vi "Plantita old.vi"() -> ()   [LabVIEW 2019]
uses:
  plantitaStates.ctl
  <vilib>/addons/control/pid/pid.llb/PID (DBL).vi
  <vilib>/addons/control/pid/NI_PID_pid.lvlib
panel:
  in  "Turbidity":bool
  in  "Sludge control":bool
  in  "Sludge valve [V]":dbl(slide)=1.5 scale=0.0..5.0
  in  "Coagulant  [V]":dbl(slide)=0.3 scale=0.0..5.0
  in  "Coagulant control":bool
  in  "Main valve [V]":dbl(slide)=2.5 scale=0.0..5.0
  in  "Flow control":bool
  out "Main valve":dbl(graph)
  in  "Shut Down":bool
  out "22 [NTU]":dbl
  out "Save File Path 2":path=path "C:/1.tdms"
  out "Settled [NTU]":dbl
  out "23 [NTU]":dbl
  out "21 [NTU]":dbl
  in  "Ripen time [s]":dbl=600.0
  in  "Backwash time [s]":dbl=600.0
  out "Last backwash":timestamp
  in  "Filtered quality target [NTU]":dbl=0.3
  out "Coagulant [mg Al/L]":dbl(graph)
  in  "Coagulant PID gains":T1={"proportional gain (Kc)"=-0.1, "integral time (Ti, min)"=33.0, "derivative time (Td, min)"=6.5} {"derivative time (Td, min)" format="%.3f"; "integral time (Ti, min)" format="%.3f"; "proportional gain (Kc)" format="%.3f"}
  out "Turbidities":dbl[][](graph)
  in  "Backwash control":bool
  out "UV 254":dbl[][](graph)
  in  "Sludge flow [L/min]":dbl=0.84
  in  "Sludge PID gains":T1={"proportional gain (Kc)"=0.07, "integral time (Ti, min)"=1.0, "derivative time (Td, min)"=0.01} {"derivative time (Td, min)" format="%.3f"; "integral time (Ti, min)" format="%.3f"; "proportional gain (Kc)" format="%.3f"}
  in  "Main PID gains":T1={"proportional gain (Kc)"=0.05, "integral time (Ti, min)"=1.0, "derivative time (Td, min)"=0.01} {"derivative time (Td, min)" format="%.3f"; "integral time (Ti, min)" format="%.3f"; "proportional gain (Kc)" format="%.3f"}
  in  "Main flow [L/min]":dbl=30.0
  out "Filter head loss":dbl
  out "Water flow value":dbl
  out "Sludge flow value":dbl
  in  "Settled quality target [NTU]":dbl=0.3
  in  "backwash [ON/OFF]":bool
  out "Sludge valve":dbl(graph)
  out "Sludge flow meter":dbl[][](graph)
  out "Filter head loss":dbl[][](graph)
  out "Main flow meter":dbl[][](graph)
  out "error out":errorcluster
  in  "Input: Seconds per data point (sec)":dbl=1.0
  in  "Start Experiment":bool
  in  "Exit":bool
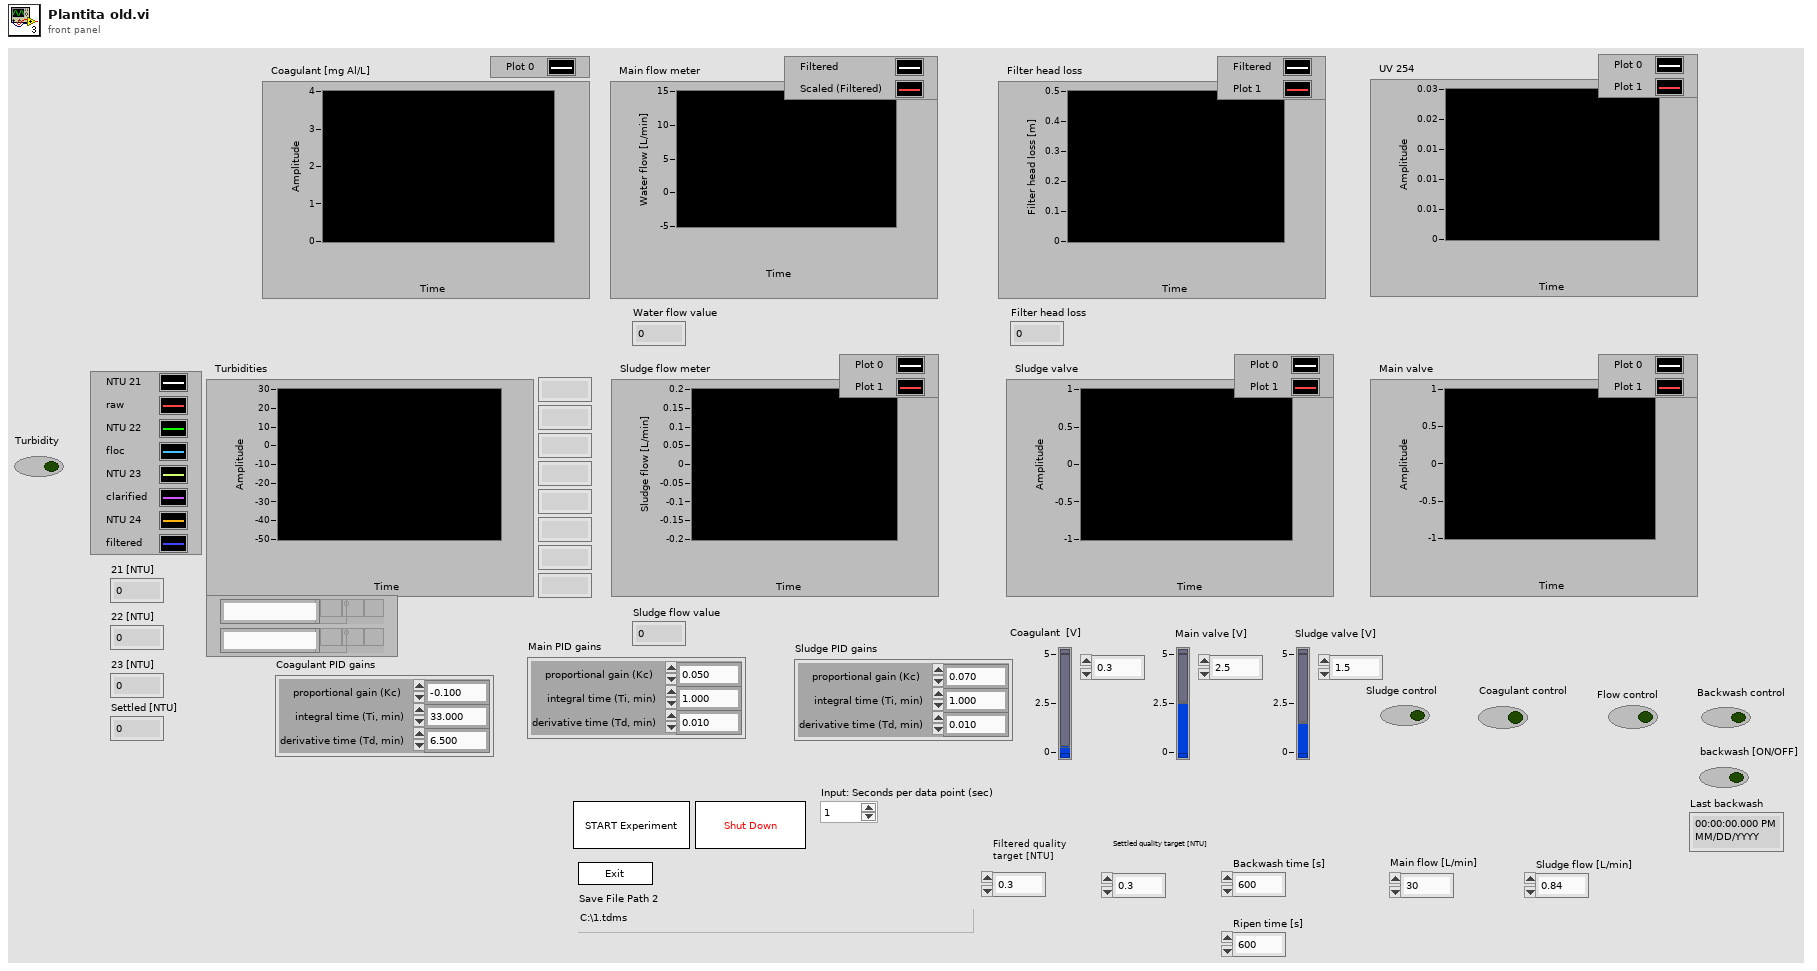
[diagram p1: front panel]
types:
  T1 = cluster{"proportional gain (Kc)":dbl, "integral time (Ti, min)":dbl, "derivative time (Td, min)":dbl}
  T2 = cluster{"Boolean <Replace Me>":bool, "String <Replace Me>":string, "Numeric <Replace Me>":dbl}
  T3 = typedef "plantitaStates.ctl" = enum16{"Initialize", "Wait for Event", "Experiment", "Exit"}
  T4 = enum16{"open", "open or create", "create or replace", "create", "open (read-only)"}
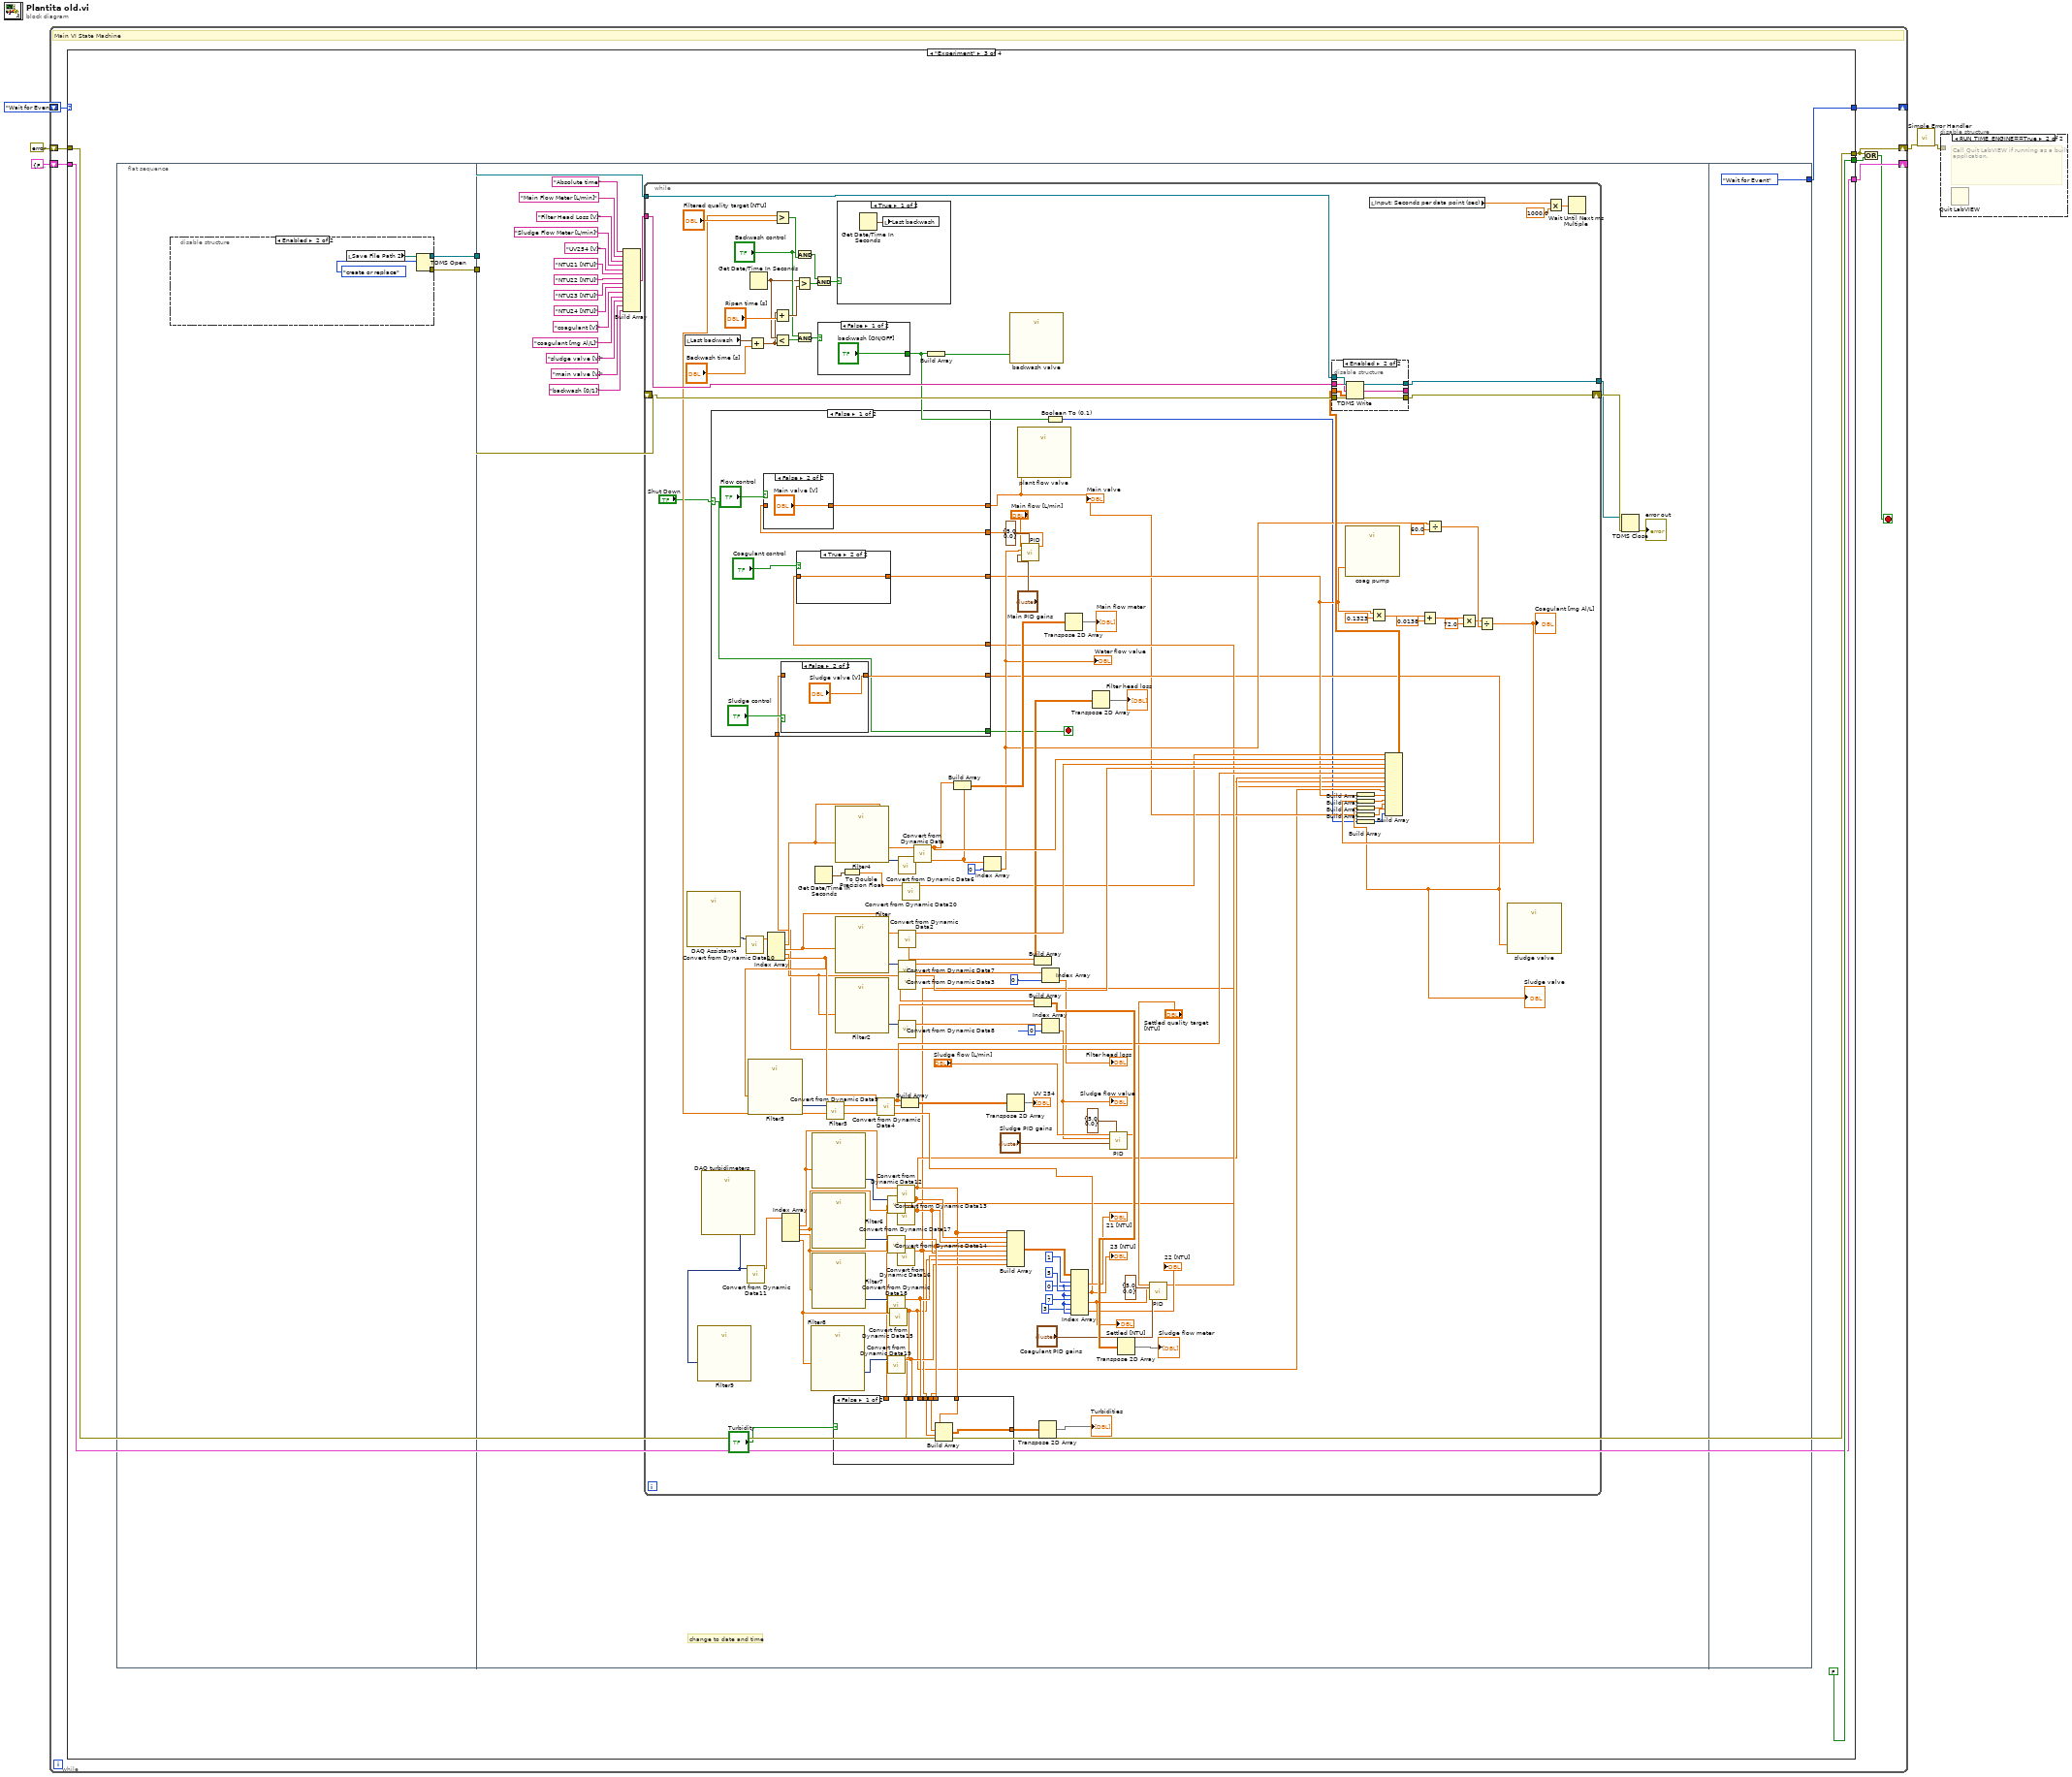
[diagram p0: block diagram]
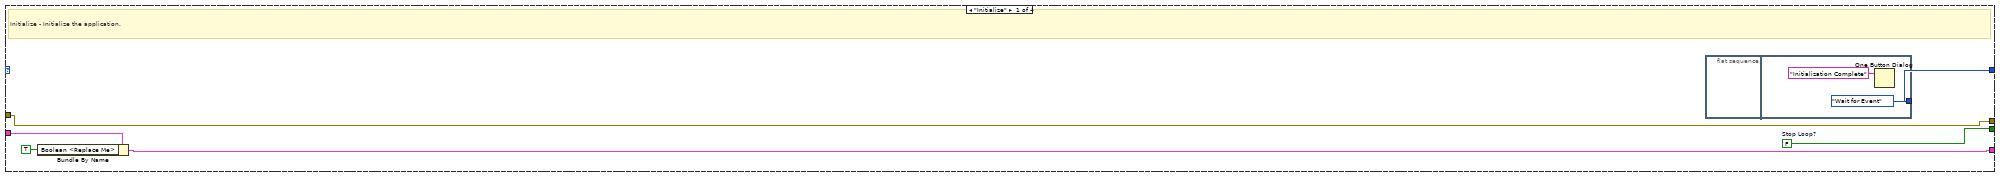
[diagram p3: hidden frame]
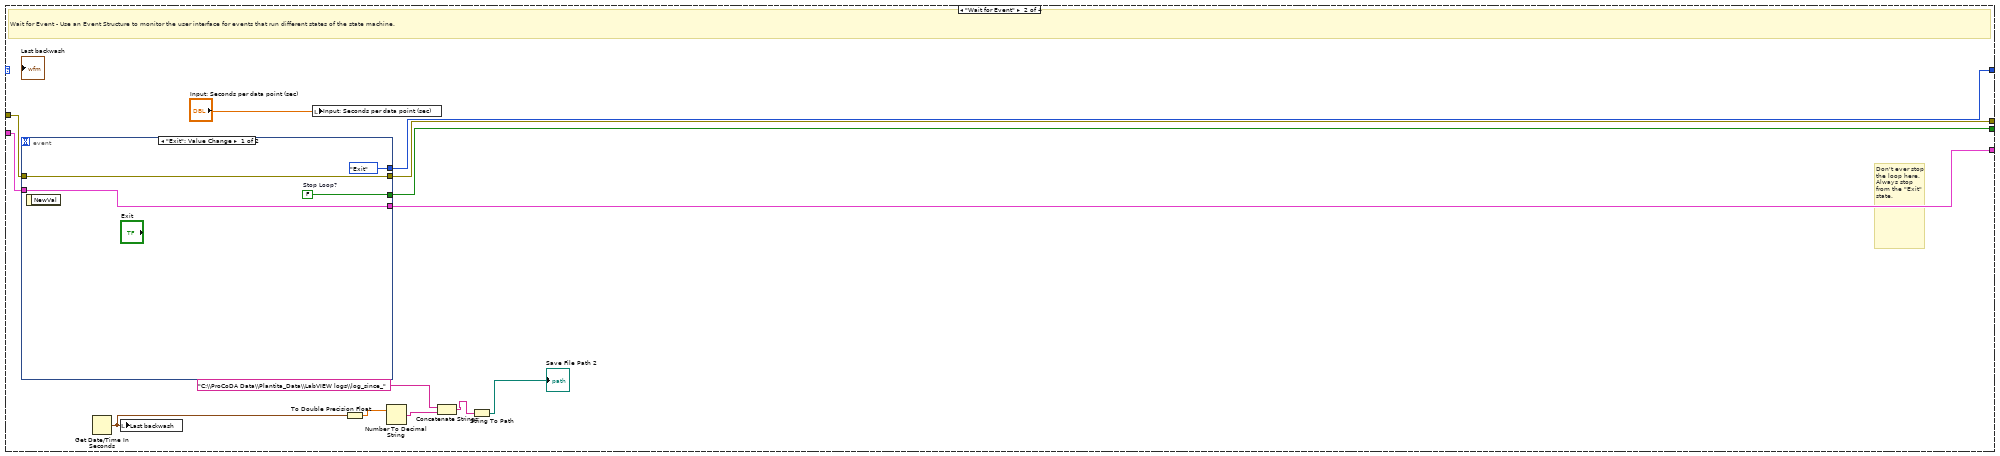
[diagram p4: hidden frame]
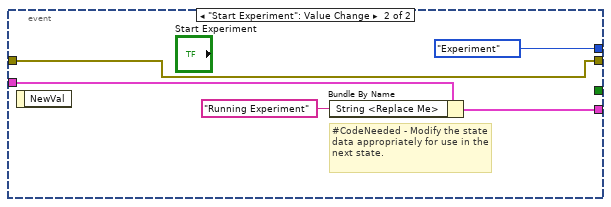
[diagram p5: hidden frame]
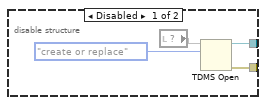
[diagram p6: hidden frame]
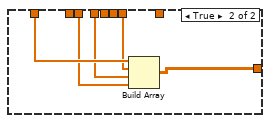
[diagram p7: hidden frame]
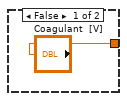
[diagram p9: hidden frame]
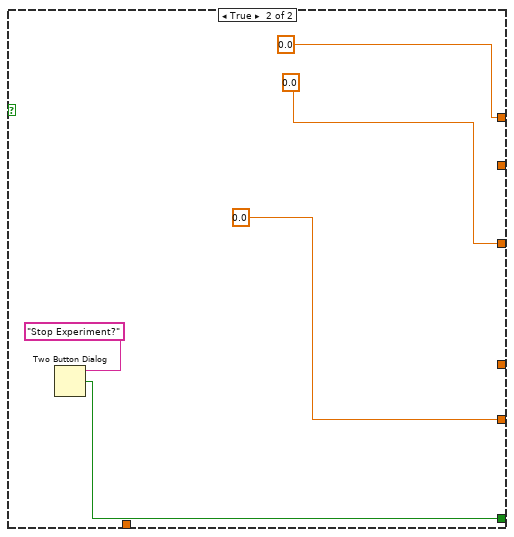
[diagram p11: hidden frame]
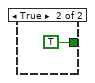
[diagram p12: hidden frame]
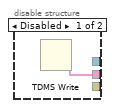
[diagram p14: hidden frame]
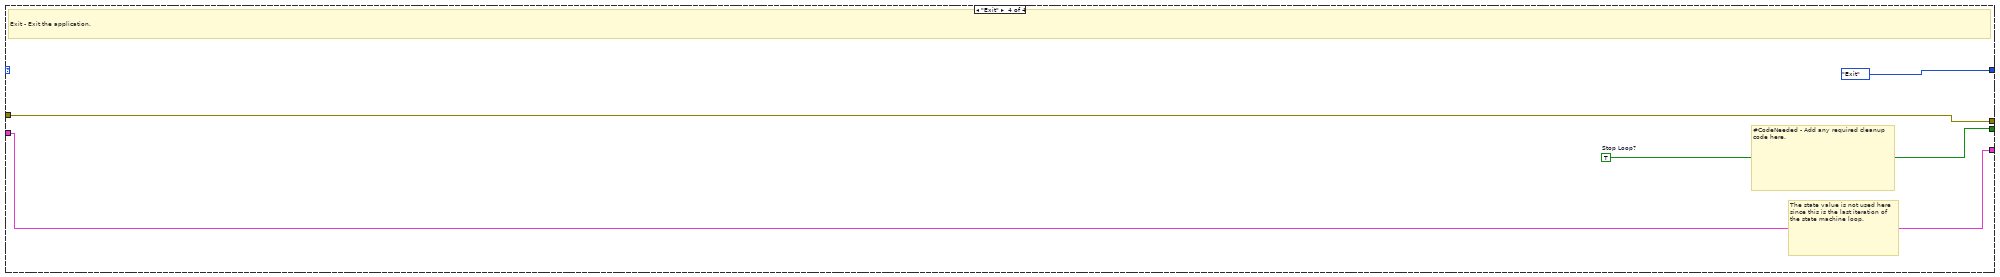
[diagram p15: hidden frame]
diagram:
  n1 = while {
    shift-right: [w12] -> _
    shift-left: plantitaStates."Wait for Event" ("Initial State") -> [w13]
    shift-right: [w10] -> _
    shift-left: T2 {"Boolean <Replace Me>"=FALSE, "String <Replace Me>"="", "Numeric <Replace Me>"=0.0} -> [w11]
    shift-right: [w6] -> w3
    shift-left: errorcluster {"status"=FALSE, "code"=0, "source"=""} ("error constant") -> [w9]
    stop <- w7 stop-if-true
    # "Main VI State Machine"
    n2 = case shown="\"Experiment\"" w13 {
      tunnel: [w14 w34 w46 plantitaStates."Exit" ("(Value Not Used)")] -> w12
      tunnel: [w19 w29 FALSE ("Stop Loop?") w252] -> w8
      tunnel: w11 -> [w18 w33 w48 w253]
      tunnel: [w17 w32 w48 w253] -> w10
      tunnel: w9 -> [w15 w31 w47 w251]
      tunnel: [w15 w30 w47 w251] -> w6
      frame "Initialize" {
        w19 = FALSE  # Stop Loop?
        # "Initialize - Initialize the application."
        n3 = Bundle By Name(cluster=w18, "Boolean <Replace Me>"=TRUE ("Replace_Me_Boolean")) -> (w17:T2)
        n4 = flat-sequence {
          tunnel: [plantitaStates."Wait for Event" ("Next State")] -> w14
          frame #0 {
          }
          frame #1 {
            n5 = One Button Dialog(message="Initialization Complete") -> ()  [unwired: 1 in, 1 out]
          }
        }
      }
      frame "Wait for Event" {
        # "Don't ever stop the loop here. Always stop from the \"Exit\" state."
        # "Wait for Event - Use an Event Structure to monitor the user interface for events that run different states of the state machine."
        n6 = event shown="[0] \"Exit\": Value Change" {
          selector: _ -> [_ _]
          dyn-events: _ -> [_ _]
          timeout: _ -> [_ _]
          tunnel: [plantitaStates."Exit" ("Next State") plantitaStates."Experiment" ("Next State")] -> w34
          tunnel: w33 -> [w37 w42]
          tunnel: [w37 w41] -> w32
          tunnel: w31 -> [w36 w39]
          tunnel: [w36 w39] -> w30
          tunnel: [w35 _] -> w29
          event "Exit": Value Change {
            w35 = FALSE  # Stop Loop?
            n7 = event-data() -> ()  [unwired: 1 in, 1 out]
          }
          event "Start Experiment": Value Change {
            # "#CodeNeeded - Modify the state data appropriately for use in the next state."
            n8 = event-data() -> ()  [unwired: 1 in, 1 out]
            n9 = Bundle By Name(cluster=w42, "String <Replace Me>"="Running Experiment" ("Running User State 1")) -> (w41:T2)
          }
        }
        n10 = Get Date/Time In Seconds() -> (seconds since 1Jan1904=w27:timestamp)
        n11 = local write "Last backwash"(w27) -> ()
        n12 = local write "Input: Seconds per data point (sec)"("Input: Seconds per data point (sec)") -> ()
        n13 = To Double Precision Float(number=w27) -> (double precision float=w25:dbl)
        n14 = Number To Decimal String(number=w25) -> (decimal integer string=w24:string)  [unwired: 1 in]
        n15 = Concatenate Strings("C:\\ProCoDA Data\\Plantita_Data\\LabVIEW logs\\log_since_", w24) -> (w23:string)
        n16 = String To Path(string=w23) -> (path=→"Save File Path 2":path)
      }
      frame "Experiment" {
        n17 = flat-sequence {
          tunnel: [w51] -> w45
          tunnel: [w50] -> w44
          tunnel: w45 -> [w77]
          tunnel: w44 -> [w79]
          tunnel: [plantitaStates."Wait for Event" ("Next State")] -> w46
          frame #0 {
            n18 = disable-structure shown="Enabled" {
              disable-tunnel: [w55 w57] -> w51
              disable-tunnel: [w54 w56] -> w50
              frame Disabled {
                n19 = local read item#-1() -> (w53)
                n20 = TDMS Open(10:T4."create or replace" ("operation (0:open)"), 11:w53) -> (0:w54:errorcluster, 3:w55:refnum<k34>)  [unwired: 5 in]
              }
              frame Enabled {
                n21 = local read "Save File Path 2"() -> (w59:path)
                n22 = TDMS Open(10:T4."create or replace" ("operation (0:open)"), 11:w59) -> (0:w56:errorcluster, 3:w57:refnum<k34>)  [unwired: 5 in]
              }
            }
          }
          frame #1 {
            # "change to date and time"
            n23 = Build Array("Absolute time", "Main Flow Meter [L/min]", "Filter Head Loss [V]", "Sludge Flow Meter [L/min]", "UV254 [V]" ("element"), "NTU21 [NTU]", "NTU22 [NTU]", "NTU23 [NTU]", "NTU24 [NTU]" ("element"), "coagulant [V]" ("element"), "coagulant [mg Al/L]" ("element"), "sludge valve [V]" ("element"), "main valve [V]" ("element"), "backwash [0/1]" ("element")) -> (w78:string[])
            n24 = while {
              shift-right: [w196] -> w75
              shift-left: w79 -> [w199]
              tunnel: w78 -> [w197]
              tunnel: w77 -> [w198]
              tunnel: [w195] -> w74
              stop <- w93 stop-if-true
              w103 = 0 ("disabled index (col)")
              n25 = local read "Last backwash"() -> (w132:timestamp)
              n26 = call "DAQ Assistant4"() -> ("data"=w168:dynamicdata)  [unwired: 17 in, 2 out]
              n27 = call "DAQ turbidimeters"() -> ("data"=w80:dynamicdata)  [unwired: 17 in, 2 out]
              n28 = call "Filter9"("Signal"=w80) -> ()  [unwired: 9 in, 2 out]
              n29 = call "Convert from Dynamic Data10"("Dynamic Data Type"=w168) -> ("Array"=w169:dbl[])  [unwired: 3 in]
              n30 = call "Convert from Dynamic Data11"("Dynamic Data Type"=w80) -> ("Array"=w159:dbl[])  [unwired: 3 in]
              n31 = Add(x=w132, y="Backwash time [s]") -> (x+y=w122:timestamp)
              n32 = Get Date/Time In Seconds() -> (seconds since 1Jan1904=w123:timestamp)
              n33 = Index Array(array=w169) -> (element #1=w167:dbl, element #2=w162:dbl, element #3=w166:dbl, element #4=w170:dbl)  [unwired: 4 in]
              n34 = call "Filter3"("Signal"=w170) -> ("Filtered Signal"=w184:dynamicdata)  [unwired: 9 in, 1 out]
              n35 = Add(x=w122, y="Ripen time [s]") -> (x+y=w130:timestamp)
              n36 = Less?(x=w123, y=w122) -> (x < y?=w124:bool)
              n37 = Index Array(array=w159) -> (element #1=w158:dbl, element #2=w154:dbl, element #3=w152:dbl, element #4=w147:dbl)  [unwired: 4 in]
              n38 = Greater?(x=w123, y=w130) -> (0:w128:bool)
              n39 = And(x="Backwash control", y=w124) -> (x .and. y?=w121:bool)
              n40 = call "Filter8"("Signal"=w147) -> ("Filtered Signal"=w148:dynamicdata)  [unwired: 9 in, 1 out]
              n41 = call "Filter5"("Signal"=w158) -> ("Filtered Signal"=w157:dynamicdata)  [unwired: 9 in, 1 out]
              n42 = call "Filter6"("Signal"=w154) -> ("Filtered Signal"=w153:dynamicdata)  [unwired: 9 in, 1 out]
              n43 = call "Filter7"("Signal"=w152) -> ("Filtered Signal"=w149:dynamicdata)  [unwired: 9 in, 1 out]
              n44 = Get Date/Time In Seconds() -> (seconds since 1Jan1904=w151:timestamp)
              n45 = case shown="False" w121 {
                tunnel: ["backwash [ON/OFF]" TRUE ("backwash [ON/OFF]")] -> w111
                frame False {
                }
                frame True {
                }
              }
              n46 = call "Convert from Dynamic Data9"("Dynamic Data Type"=w184) -> ("Array"=w179:dbl[])  [unwired: 3 in]
              n47 = call "Filter4"("Signal"=w167) -> ("Filtered Signal"=w193:dynamicdata)  [unwired: 9 in, 1 out]
              n48 = call "Filter"("Signal"=w162) -> ("Filtered Signal"=w188:dynamicdata)  [unwired: 9 in, 1 out]
              n49 = call "Filter2"("Signal"=w166) -> ("Filtered Signal"=w185:dynamicdata)  [unwired: 9 in, 1 out]
              n50 = To Double Precision Float(number=w151) -> (double precision float=w150:dbl)
              n51 = call "Convert from Dynamic Data4"("Dynamic Data Type"=w170) -> ("Array"=w180:dbl[])  [unwired: 3 in]
              n52 = call "Convert from Dynamic Data13"("Dynamic Data Type"=w157) -> ("Array"=w91:dbl[])  [unwired: 3 in]
              n53 = call "Convert from Dynamic Data14"("Dynamic Data Type"=w153) -> ("Array"=w90:dbl[])  [unwired: 3 in]
              n54 = call "Convert from Dynamic Data18"("Dynamic Data Type"=w149) -> ("Array"=w89:dbl[])  [unwired: 3 in]
              n55 = call "Convert from Dynamic Data19"("Dynamic Data Type"=w148) -> ("Array"=w88:dbl[])  [unwired: 3 in]
              n56 = call "Convert from Dynamic Data15"("Dynamic Data Type"=w147) -> ("Array"=w84:dbl[])  [unwired: 3 in]
              n57 = call "Convert from Dynamic Data12"("Dynamic Data Type"=w158) -> ("Array"=w87:dbl[])  [unwired: 3 in]
              n58 = call "Convert from Dynamic Data17"("Dynamic Data Type"=w154) -> ("Array"=w86:dbl[])  [unwired: 3 in]
              n59 = call "Convert from Dynamic Data16"("Dynamic Data Type"=w152) -> ("Array"=w85:dbl[])  [unwired: 3 in]
              n60 = case shown="False" "Turbidity" {
                tunnel: [w207 w212] -> w92
                tunnel: w91 -> [_ w211]
                tunnel: w90 -> [_ w210]
                tunnel: w89 -> [_ w209]
                tunnel: w88 -> [_ w208]
                tunnel: w87 -> [w206 _]
                tunnel: w86 -> [w205 _]
                tunnel: w85 -> [w204 _]
                tunnel: w84 -> [w203 _]
                frame False {
                  n61 = Build Array "Build Array"(w206, w205, w204, w203) -> (w207:dbl[][])
                }
                frame True {
                  n62 = Build Array "Build Array"(w211, w210, w209, w208) -> (w212:dbl[][])
                }
              }
              n63 = call "Convert from Dynamic Data6"("Dynamic Data Type"=w193) -> ("Array"=w177:dbl[])  [unwired: 3 in]
              n64 = call "Convert from Dynamic Data7"("Dynamic Data Type"=w188) -> ("Array"=w172:dbl[])  [unwired: 3 in]
              n65 = call "Convert from Dynamic Data8"("Dynamic Data Type"=w185) -> ("Array"=w171:dbl[])  [unwired: 3 in]
              n66 = call "Convert from Dynamic Data2"("Dynamic Data Type"=w162) -> ("Array"=w189:dbl[])  [unwired: 3 in]
              n67 = call "Convert from Dynamic Data3"("Dynamic Data Type"=w166) -> ("Array"=w183:dbl[])  [unwired: 3 in]
              n68 = Build Array(w180, w179) -> (w178:dbl[][])
              n69 = call "Convert from Dynamic Data20"("Dynamic Data Type"=w150) -> ("Array"=w109:dbl[])  [unwired: 3 in]
              n70 = call "Convert from Dynamic Data"("Dynamic Data Type"=w167) -> ("Array"=w190:dbl[])  [unwired: 3 in]
              n71 = Build Array(w111) -> (w112:bool[])
              n72 = Build Array(w190, w177) -> (w191:dbl[][])
              n73 = Index Array(array=w177, index=0) -> (element=w139:dbl)
              "Water flow value" <- w139
              n74 = Transpose 2D Array(2D array=w178) -> (transposed array=→"UV 254":dbl[][])
              n75 = Build Array "Build Array"(w87, w91, w86, w90, w85, w89, w84, w88) -> (w120:dbl[][])
              n76 = call "backwash valve"("data"=w112) -> ()  [unwired: 17 in, 2 out]
              n77 = call-poly <vilib>:"PID.vi"("output range"=cluster{"output high":dbl, "output low":dbl} {"output high"=5.0, "output low"=0.0}, "PID gains"="Main PID gains", "process variable"=w139, "setpoint"="Main flow [L/min]") -> ("output"=w99:dbl)  [unwired: 6 in, 1 out]
              n78 = Build Array(w189, w172) -> (w186:dbl[][])
              n79 = Build Array(w183, w171) -> (w182:dbl[][])
              n80 = Transpose 2D Array(2D array=w92) -> (transposed array=→"Turbidities":dbl[][])
              n81 = Index Array(array=w172, index=0) -> (element=→"Filter head loss":dbl)
              n82 = Index Array(array=w171, index=0) -> (element=w156:dbl)
              "Sludge flow value" <- w156
              n83 = Boolean To (0,1)(Boolean=w111) -> (0, 1=w81:i16)
              n84 = Transpose 2D Array(2D array=w191) -> (transposed array=→"Main flow meter":dbl[][])
              n85 = Index Array(array=w120, index (row) #1=1 ("index (row)"), index (col) #1=w103, index (row) #2=5 ("disabled index (row)"), index (col) #2=w103, index (row) #3=7 ("disabled index (row)"), index (col) #3=w103, index (row) #4=3 ("disabled index (row)"), index (col) #4=w103) -> (element #1=→"21 [NTU]":dbl, element #2=w113:dbl, element #3=w115:dbl, element #4=→"22 [NTU]":dbl)
              "23 [NTU]" <- w113
              "Settled [NTU]" <- w115
              n86 = Greater?(x=w113, y="Filtered quality target [NTU]") -> (0:w134:bool)
              n87 = And(x="Backwash control", y=w134) -> (x .and. y?=w126:bool)
              n88 = And(x=w126, y=w128) -> (x .and. y?=w127:bool)
              n89 = case shown="True" w127 {
                frame True {
                  n90 = Get Date/Time In Seconds() -> (seconds since 1Jan1904=w236:timestamp)
                  n91 = local write "Last backwash"(w236) -> ()
                }
                frame False {
                }
              }
              n92 = Transpose 2D Array(2D array=w186) -> (transposed array=→"Filter head loss":dbl[][])
              n93 = call-poly <vilib>:"PID.vi"("output range"=cluster{"output high":dbl, "output low":dbl} {"output high"=5.0, "output low"=0.0}, "PID gains"="Sludge PID gains", "process variable"=w156, "setpoint"="Sludge flow [L/min]") -> ("output"=w96:dbl)  [unwired: 6 in, 1 out]
              n94 = Transpose 2D Array(2D array=w182) -> (transposed array=→"Sludge flow meter":dbl[][])
              n95 = call-poly <vilib>:"PID.vi"("output range"=cluster{"output high":dbl, "output low":dbl} {"output high"=5.0, "output low"=0.0}, "PID gains"="Coagulant PID gains", "process variable"=w115, "setpoint"="Settled quality target [NTU]") -> ("output"=w97:dbl)  [unwired: 6 in, 1 out]
              n96 = case shown="False" "Shut Down" {
                selector: "Shut Down" -> [w213 _]
                tunnel: w99 -> [w221 _]
                tunnel: [w220 0.0 ("Main valve [V] 2")] -> w94
                tunnel: [w218 0.0 ("Main valve [V] 2")] -> w98
                tunnel: w97 -> [w217 _]
                tunnel: w96 -> [w215 _]
                tunnel: [w214 0.0 ("Main valve [V] 2")] -> w95
                tunnel: [w213 w229] -> w93
                frame False {
                  n97 = case shown="False" "Flow control" {
                    tunnel: [w227 "Main valve [V]"] -> w220
                    tunnel: w221 -> [w227 _]
                    frame True {
                    }
                    frame False {
                    }
                  }
                  n98 = case shown="False" "Sludge control" {
                    tunnel: [w223 "Sludge valve [V]"] -> w214
                    tunnel: w215 -> [w223 _]
                    frame True {
                    }
                    frame False {
                    }
                  }
                  n99 = case shown="True" "Coagulant control" {
                    tunnel: w217 -> [_ w226]
                    tunnel: ["Coagulant  [V]" w226] -> w218
                    frame False {
                    }
                    frame True {
                    }
                  }
                }
                frame True {
                  n100 = Two Button Dialog(message="Stop Experiment?") -> (T button?=w229:bool)  [unwired: 2 in]
                }
              }
              "Sludge valve" <- w95
              "Main valve" <- w94
              n101 = call "plant flow valve"("data"=w94) -> ()  [unwired: 17 in, 2 out]
              n102 = call "coag pump"("data"=w98) -> ()  [unwired: 17 in, 2 out]
              n103 = Build Array(w98) -> (w104:dbl[])
              n104 = Build Array(w95) -> (w106:dbl[])
              n105 = Build Array(w94) -> (w107:dbl[])
              n106 = Build Array(w81) -> (w108:i16[])
              n107 = local read "Input: Seconds per data point (sec)"() -> (w200:dbl)
              n108 = Multiply(x=w98, y=0.1323) -> (x*y=w142:dbl)
              n109 = Add(x=w142, y=0.0138) -> (x+y=w137:dbl)
              n110 = Divide(x=w139, y=60.0) -> (x/y=w138:dbl)
              n111 = Multiply(x=w137, y=72.0) -> (x*y=w136:dbl)
              n112 = Divide(x=w136, y=w138) -> (x/y=w110:dbl)
              "Coagulant [mg Al/L]" <- w110
              n113 = Build Array(w110) -> (w105:dbl[])
              n114 = Build Array(w109, w190, w189, w183, w180, w87, w86, w85, w84, w104, w105, w106, w107, w108) -> (w194:dbl[][])
              n115 = disable-structure shown="Enabled" {
                disable-tunnel: [w238 w245] -> _
                disable-tunnel: w199 -> [_ w249]
                disable-tunnel: [_ w248] -> w196
                disable-tunnel: [_ w247] -> w195
                disable-tunnel: w198 -> [_ w246]
                disable-tunnel: w197 -> [_ w244]
                disable-tunnel: w194 -> [_ w243]
                frame Disabled {
                  n116 = TDMS Write(7:w238) -> (0:w241:refnum<k34>, 4:w242:refnum<k34>, 9:w237:waveform(dbl)[], 11:w240:errorcluster, 15:w239:errorcluster)  [unwired: 2 in, 2 out]
                }
                frame Enabled {
                  n117 = TDMS Write(0:w246, 7:w244, 9:w243, 11:w249) -> (4:w247:refnum<k34>, 8:w245:string[], 15:w248:errorcluster)  [unwired: 2 in, 1 out]
                }
              }
              n118 = call "sludge valve"("data"=w95) -> ()  [unwired: 17 in, 2 out]
              n119 = Multiply(x=w200, y=1000.0) -> (x*y=w202:dbl)
              n120 = Wait Until Next ms Multiple(millisecond multiple=w202) -> ()  [unwired: 1 out]
            }
            n121 = TDMS Close(8:w75, 11:w74) -> (0:→"error out":errorcluster)  [unwired: 1 out]
          }
          frame #2 {
          }
        }
      }
      frame "Exit" {
        w252 = TRUE  # Stop Loop?
        # "#CodeNeeded - Add any required cleanup code here."
        # "The state value is not used here since this is the last iteration of the state machine loop."
        # "Exit - Exit the application."
      }
    }
    n122 = Or(x=w6, y=w8) -> (x .or. y?=w7:bool)
  }
  n123 = call <vilib>:"Simple Error Handler.vi"("error in (no error)"=w3) -> ("error out"=w2:errorcluster)  [unwired: 4 in, 4 out]
  n124 = disable-structure shown="RUN_TIME_ENGINE==True" {
    disable-tunnel: w2 -> [_ _]
    frame condition #0 (active) {
    }
    frame condition #1 {
      # "Call Quit LabVIEW if running as a built application."
      n125 = Quit LabVIEW() -> ()  [unwired: 1 in]
    }
  }
